vi "gpio_exp02.vi"() -> ()   [LabVIEW 2014]
uses:
  usr/local/lib/libgpio_exp02.dll
panel:
  out "Status 4":bool
  out "Status 3":bool
  out "Status 2":bool
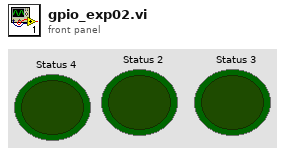
[diagram p1: front panel]
types:
  T1 = enum8{"INPUT", "OUTPUT", "PWM_OUTPUT", "GPIO_CLOCK", "SOFT_PWM_OUTPUT", "SOFT_TONE_OUTPUT", "PWM_TONE_OUTPUT"}
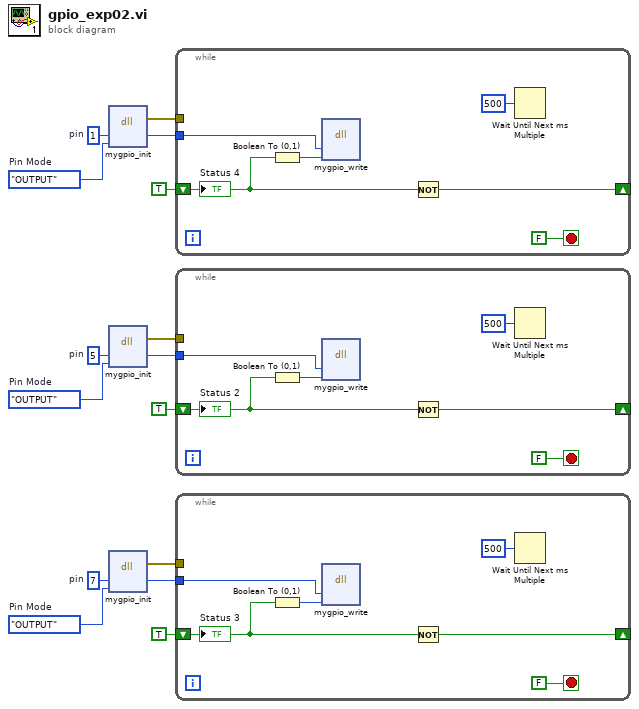
[diagram p0: block diagram]
diagram:
  w1 = T1."OUTPUT"  # Pin Mode
  w4 = u8 1  # pin
  w6 = T1."OUTPUT"  # Pin Mode
  w9 = u8 7  # pin
  w15 = T1."OUTPUT"  # Pin Mode
  w12 = u8 5  # pin
  n1 = dll-call lib="usr/local/lib/libgpio_exp02.*" fn="mygpio_init"("pin"=w4, "mode"=w1) -> (error out=w3:errorcluster, "pin"=w5:u8)  [unwired: 5 in, 1 out]
  n2 = dll-call lib="usr/local/lib/libgpio_exp02.*" fn="mygpio_init"("pin"=w12, "mode"=w15) -> (error out=w13:errorcluster, "pin"=w11:u8)  [unwired: 5 in, 1 out]
  n3 = dll-call lib="usr/local/lib/libgpio_exp02.*" fn="mygpio_init"("pin"=w9, "mode"=w6) -> (error out=w8:errorcluster, "pin"=w10:u8)  [unwired: 5 in, 1 out]
  n4 = while {
    tunnel: w3 -> [_]
    shift-right: [w17] -> _
    shift-left: TRUE -> [w20]
    tunnel: w5 -> [w16]
    stop <- FALSE stop-if-true
    n5 = Boolean To (0,1)(Boolean=w20) -> (0, 1=w21:i16)
    n6 = dll-call lib="usr/local/lib/libgpio_exp02.*" fn="mygpio_write"("pin"=w16, "state"=w21) -> ()  [unwired: 6 in, 2 out]
    n7 = Not(x=w20) -> (.not. x?=w17:bool)
    n8 = Wait Until Next ms Multiple(millisecond multiple=u32 500) -> ()  [unwired: 1 out]
    "Status 4" <- w20
  }
  n9 = while {
    tunnel: w13 -> [_]
    shift-right: [w23] -> _
    shift-left: TRUE -> [w26]
    tunnel: w11 -> [w22]
    stop <- FALSE stop-if-true
    n10 = Boolean To (0,1)(Boolean=w26) -> (0, 1=w27:i16)
    n11 = dll-call lib="usr/local/lib/libgpio_exp02.*" fn="mygpio_write"("pin"=w22, "state"=w27) -> ()  [unwired: 6 in, 2 out]
    n12 = Not(x=w26) -> (.not. x?=w23:bool)
    n13 = Wait Until Next ms Multiple(millisecond multiple=u32 500) -> ()  [unwired: 1 out]
    "Status 2" <- w26
  }
  n14 = while {
    tunnel: w8 -> [_]
    shift-right: [w29] -> _
    shift-left: TRUE -> [w32]
    tunnel: w10 -> [w28]
    stop <- FALSE stop-if-true
    n15 = Boolean To (0,1)(Boolean=w32) -> (0, 1=w33:i16)
    n16 = dll-call lib="usr/local/lib/libgpio_exp02.*" fn="mygpio_write"("pin"=w28, "state"=w33) -> ()  [unwired: 6 in, 2 out]
    n17 = Not(x=w32) -> (.not. x?=w29:bool)
    n18 = Wait Until Next ms Multiple(millisecond multiple=u32 500) -> ()  [unwired: 1 out]
    "Status 3" <- w32
  }
